vi "Self-Test.vi"(8 "error in (no error)":errorcluster, 11 "VISA resource name":refnum<visa-resource-name>) -> (0 "error out":errorcluster, 1 "Self-Test Response":string, 2 "Self-Test Error":u32, 3 "VISA resource name out":refnum<visa-resource-name>)   [LabVIEW 2015, in "Agilent 428X Series.lvlib"]
doc: "This VI causes the instrument to perform a self-test and returns the results. A numeric indicator indicates if the instrument passed all self-tests, and a string indicator contains the instrument's reponse. If a self test is not supported, the VI returns a warning code."
uses:
  Agilent 428X Series.lvlib
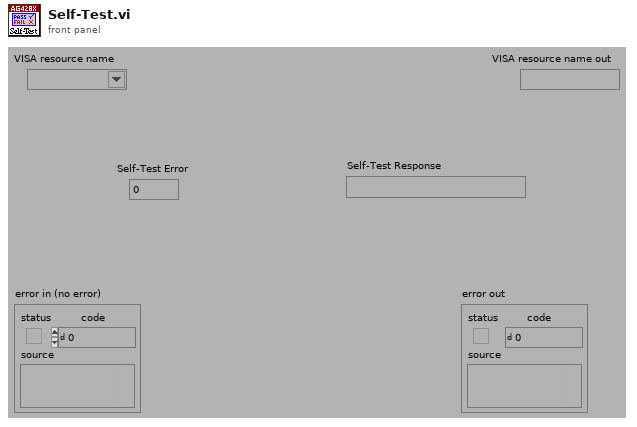
[diagram p1: front panel]
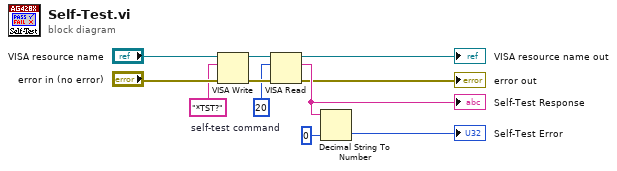
[diagram p0: block diagram]
diagram:
  w5 = "*TST?"  # self-test command
  n1 = VISA Write(VISA resource name="VISA resource name", write buffer=w5, error in (no error)="error in (no error)") -> (VISA resource name out=w2:refnum<visa-resource-name>, error out=w4:errorcluster)  [unwired: 1 out]
  n2 = VISA Read(VISA resource name=w2, byte count=u32 20, error in (no error)=w4) -> (VISA resource name out=→"VISA resource name out":refnum<visa-resource-name>, read buffer=w11:string, error out=→"error out":errorcluster)  [unwired: 1 out]
  "Self-Test Response" <- w11
  n3 = Decimal String To Number(string=w11, default (0L)=u32 0) -> (number=→"Self-Test Error":u32)  [unwired: 1 in, 1 out]
